vi "RFH-allign_data.vi"(7 "Xi":dbl[](array[numeric]), 10 "Common Format":T1) -> (2 "Common Format alligned":T1)   [LabVIEW 2020, in "RFH-Reflection_File_Handler.lvlib"]
uses:
  RFH-Reflection_File_Handler.lvlib
  RFH-common_data_format.ctl
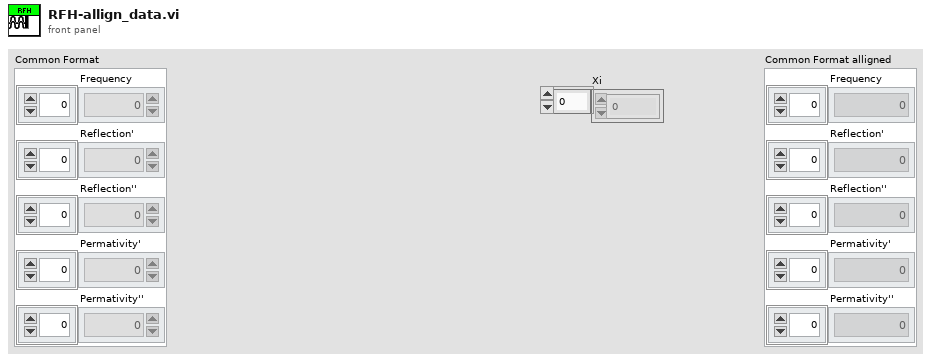
[diagram p1: front panel]
types:
  T1 = typedef "RFH-Reflection_File_Handler.lvlib/RFH-common_data_format.ctl" = cluster{"Frequency":dbl[], "Reflection'":dbl[], "Reflection''":dbl[], "Permativity'":dbl[], "Permativity''":dbl[]}
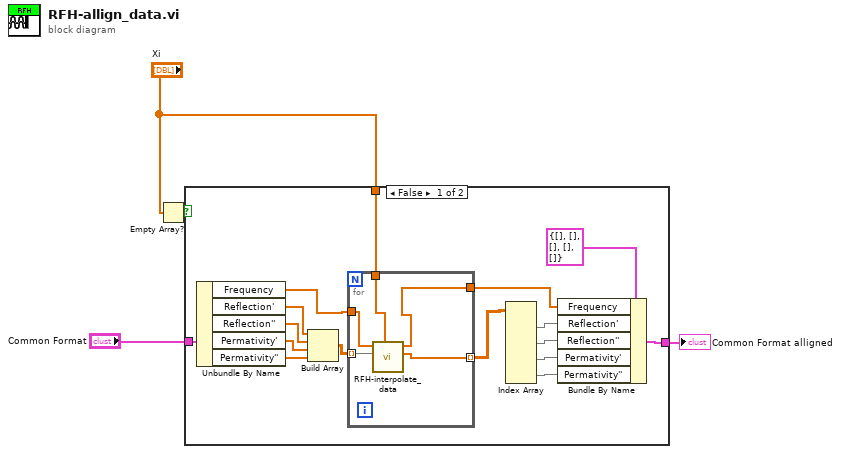
[diagram p0: block diagram]
diagram:
  n1 = Empty Array?(array="Xi") -> (empty?=w3:bool)
  n2 = case shown="False" w3 {
    tunnel: "Xi" -> [w16 _]
    tunnel: "Common Format" -> [w15 w26]
    tunnel: [w8 w26] -> w1
    frame False {
      n3 = Unbundle By Name(w15) -> ("Frequency"=w17:dbl[], "Reflection'"=w20:dbl[], "Reflection''"=w19:dbl[], "Permativity'"=w7:dbl[], "Permativity''"=w6:dbl[])
      n4 = Build Array(w20, w19, w7, w6) -> (w18:dbl[][])
      n5 = for {
        tunnel: w18 -> [w25] mode=indexing
        tunnel: w17 -> [w24]
        tunnel: w16 -> [w23]
        tunnel: [w21] -> w10 mode=indexing
        tunnel: [w22] -> w9
        n6 = call "RFH-interpolate_data.vi"("Xi"=w23, "data"=w25, "Frequency"=w24) -> ("data out"=w21:dbl[], "Frequency out"=w22:dbl[])  [unwired: 7 in]
      }
      n7 = Index Array(array=w10) -> (element #1=w11:dbl[], element #2=w12:dbl[], element #3=w13:dbl[], element #4=w14:dbl[])  [unwired: 8 in]
      n8 = Bundle By Name(cluster=T1 {"Frequency"=[], "Reflection'"=[], "Reflection''"=[], "Permativity'"=[], "Permativity''"=[]} ("Common Format"), "Frequency"=w9, "Reflection'"=w11, "Reflection''"=w12, "Permativity'"=w13, "Permativity''"=w14) -> (w8:T1)
    }
    frame True {
    }
  }
  "Common Format alligned" <- w1
